vi "read_all_positions.vi"(10 "error in":errorcluster, 11 "VISA Refnum in":refnum<visa-resource-name>) -> (0 "z position":dbl format="%.2f", 1 "y position":dbl format="%.2f", 2 "x position":dbl format="%.2f", 3 "r position":dbl format="%.2f", 4 "error out":errorcluster, 5 "VISA Handle out":refnum<visa-resource-name>)   [LabVIEW 2025]
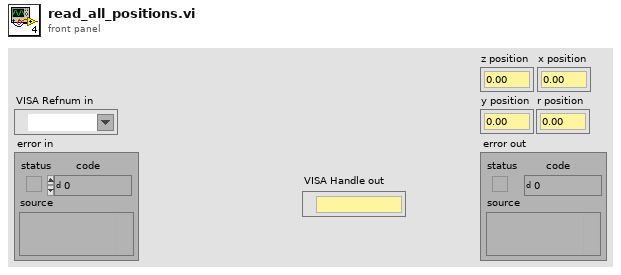
[diagram p1: front panel]
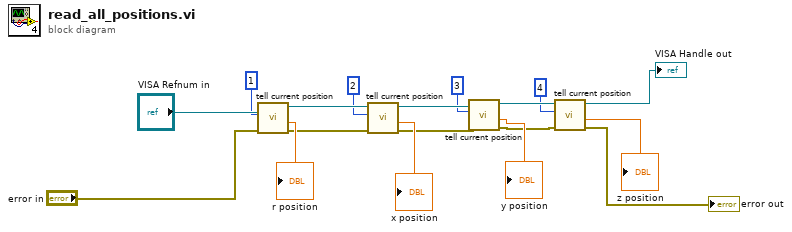
[diagram p0: block diagram]
diagram:
  n1 = call <userlib>:"tell current position.vi"("error in"="error in", "Axis in"=1, "VISA Handle in"="VISA Refnum in") -> ("error out"=w4:errorcluster, "Current position (units)"=→"r position":dbl, "VISA Handle out"=w17:refnum<visa-resource-name>)  [unwired: 2 in, 2 out]
  n2 = call <userlib>:"tell current position.vi"("error in"=w4, "Axis in"=2, "VISA Handle in"=w17) -> ("error out"=w3:errorcluster, "Current position (units)"=→"x position":dbl, "VISA Handle out"=w16:refnum<visa-resource-name>)  [unwired: 2 in, 2 out]
  n3 = call <userlib>:"tell current position.vi"("error in"=w3, "Axis in"=3, "VISA Handle in"=w16) -> ("error out"=w2:errorcluster, "Current position (units)"=→"y position":dbl, "VISA Handle out"=w15:refnum<visa-resource-name>)  [unwired: 2 in, 2 out]
  n4 = call <userlib>:"tell current position.vi"("error in"=w2, "Axis in"=4, "VISA Handle in"=w15) -> ("error out"=→"error out":errorcluster, "Current position (units)"=→"z position":dbl, "VISA Handle out"=→"VISA Handle out":refnum<visa-resource-name>)  [unwired: 2 in, 2 out]
